vi "CSM - Query Internal Data Names By API String.vi"(6 "Response Timeout(5000ms)":i32=5000, 7 "Current Module(\"\" to generate a ID)":string, 8 "Error In (no error)":errorcluster, 9 "Target Module":string="A") -> (0 "error out":errorcluster, 3 "Configurations":string[](array[string]))   [LabVIEW 2017, in "API String Arguments Support.lvlib"]
uses:
  API String Arguments Support.lvlib
  3795495c-8fc1-4c3f-b539-16526106a5d1.vi
  _Support/Convert API String Arguments to Data(variant).vi
  <userlib>/_NEVSTOP/Communicable State Machine(CSM)/Communicable State Machine.lvlib
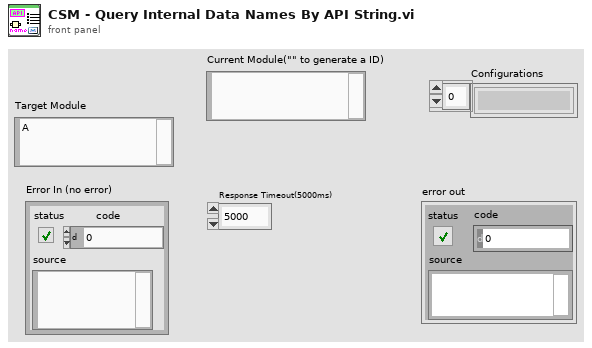
[diagram p1: front panel]
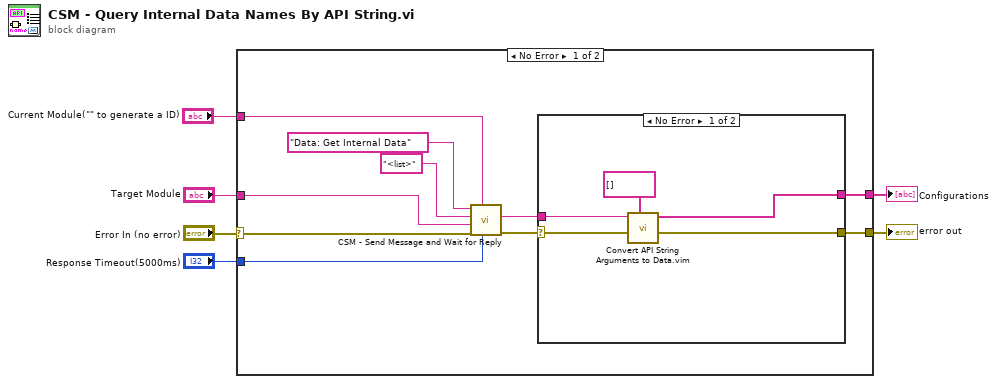
[diagram p0: block diagram]
diagram:
  n1 = case shown="No Error" "Error In (no error)" {
    selector: "Error In (no error)" -> [w11 w23]
    tunnel: "Response Timeout(5000ms)" -> [w15 _]
    tunnel: [w12 w23] -> w5
    tunnel: [w9 _] -> w3
    tunnel: "Target Module" -> [w8 _]
    tunnel: "Current Module(\"\" to generate a ID)" -> [w7 _]
    frame No Error {
      n2 = call <userlib>:"CSM - Send Message and Wait for Reply.vi"("Response Timeout(-2 using Global Settings)"=w15, "Current Module(\"\" to generate a ID)"=w7, "Error In (no error)"=w11, "Target Module"=w8, "Arguments (\"\")"="<list>" ("Name(\"\" to use uuid)"), "State"="Data: Get Internal Data") -> ("error out"=w13:errorcluster, "Response"=w14:string)  [unwired: 3 in, 1 out]
      n3 = case shown="No Error" w13 {
        selector: w13 -> [w20 w22]
        tunnel: w14 -> [w21 _]
        tunnel: [w19 w22] -> w12
        tunnel: [w17 _] -> w9
        frame No Error {
          n4 = call "Convert API String Arguments to Data.vim"("Type"=string[] [] ("Name(\"\" to use uuid)"), "error in (no error)"=w20, "String"=w21) -> ("error"=w19:errorcluster, "Data"=w17:string[])  [unwired: 5 in]
        }
        frame Error {
        }
      }
    }
    frame Error {
    }
  }
  "error out" <- w5
  "Configurations" <- w3
